vi "Process Lines From File.vi"() -> ()   [LabVIEW 2023]
doc: "This VI illustrates the use of a sequence of string Stream channels to process text. The sequence of channel-connected subVIs creates a highly parallel pipeline architecture."
uses:
  <extravilib>/ChannelInstances/Stream-str/Read.vi
  <extravilib>/ChannelInstances/Stream-str/Read With Abort.vi
  <extravilib>/ChannelInstances/Stream-str/EndpointRead.vi
  <extravilib>/ChannelInstances/Stream-str/Instantiate.vi
  <extravilib>/ChannelInstances/Stream-str/)Channel.vi
  <resource>/ChannelSupport/_ChannelSupport/WaitIfNeeded.vi
  <extravilib>/ChannelInstances/Stream-str.lvlib
panel:
  out "total words":i32
  out "words":string[](array[string])
  in  "pattern":string="[vw]"
  in  "file path":path
  # "Overview: Demonstrates the use of the Stream channel in processing strings from a text file. This VI reads a text file specified by file path and filters lines based on pattern. The chosen lines are processed to produce a list of all the unique words in the lines, sorted alphabetically.\n\nInstructions:\n1. Run the VI (which will use a default text file).  The output word list contains 38 unique words beginning with \"A\" and ending with \"with\".\n2. Enter your own settings for file path and pattern (use the syntax for the Match Pattern function). Run the VI again.\n3. See block diagram."
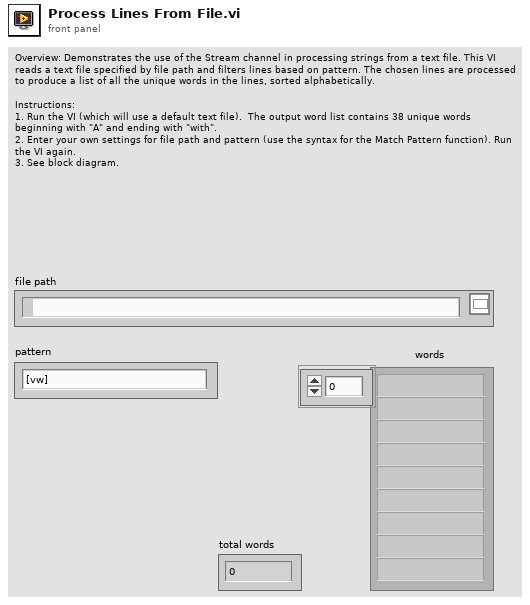
[diagram p1: front panel]
types:
  T1 = typedef "Stream-str.lvlib/)Channel.ctl" = refnum<queue>
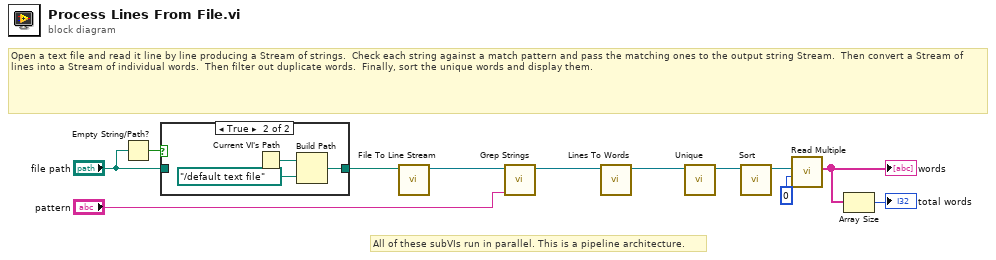
[diagram p0: block diagram]
diagram:
  # "All of these subVIs run in parallel. This is a pipeline architecture."
  # "Open a text file and read it line by line producing a Stream of strings.  Check each string against a match pattern and pass the matching ones to the output string Stream.  Then convert a Stream of lines into a Stream of individual words.  Then filter out duplicate words.  Finally, sort the unique words and display them."
  n1 = Empty String/Path?(string/path="file path") -> (empty?=w10:bool)
  n2 = case shown="True" w10 {
    tunnel: [w13 w16] -> w9
    tunnel: "file path" -> [w13 _]
    frame False {
    }
    frame True {
      n3 = Current VI's Path() -> (path=w15:path)
      n4 = Build Path(base path=w15, name or relative path=path "../default text file") -> (appended path=w16:path)
    }
  }
  n5 = call "File To Line Stream.vi"("file path"=w9) -> ("lines"=w12:T1)  [unwired: 10 in]
  n6 = call "Grep Strings.vi"("match pattern"="pattern", "strings in"=w12) -> ("strings out"=w7:T1)  [unwired: 9 in]
  n7 = call "Lines To Words.vi"("lines in"=w7) -> ("words out"=w6:T1)  [unwired: 10 in]
  n8 = call "Unique.vi"("strings in"=w6) -> ("unique strings out"=w5:T1)  [unwired: 10 in]
  n9 = call "Sort.vi"("strings in"=w5) -> ("sorted strings out"=w4:T1)  [unwired: 10 in]
  n10 = call <extravilib>:"Read Multiple.vi"("number to read (-1, available)"=0, "channel"=w4) -> ("elements"=w2:string[])  [unwired: 6 in, 3 out]
  "words" <- w2
  n11 = Array Size(array=w2) -> (size(s)=→"total words":i32)
